vi "ReadMDF.vi"() -> (2 "Number of Waypoints Read":i32, 3 "MDF Array out":T2)   [LabVIEW 2010]
uses:
  4-High Neurons/MDFArray.ctl
  4-High Neurons/MissionDefinitionFile.ctl
panel:
  in  "MissionDefinition":T1={"Waypoint #"=2.0, "X (waypoint)"=0.0, "Y (waypoint)"=0.0, "Vel (desired)"=0.0, "Dwell Time"=0.0, "Behavior"=enum."OpenFieldTransit", "Expand1"=0.0, "Expand2"=0.0, "Expand3"=0.0}
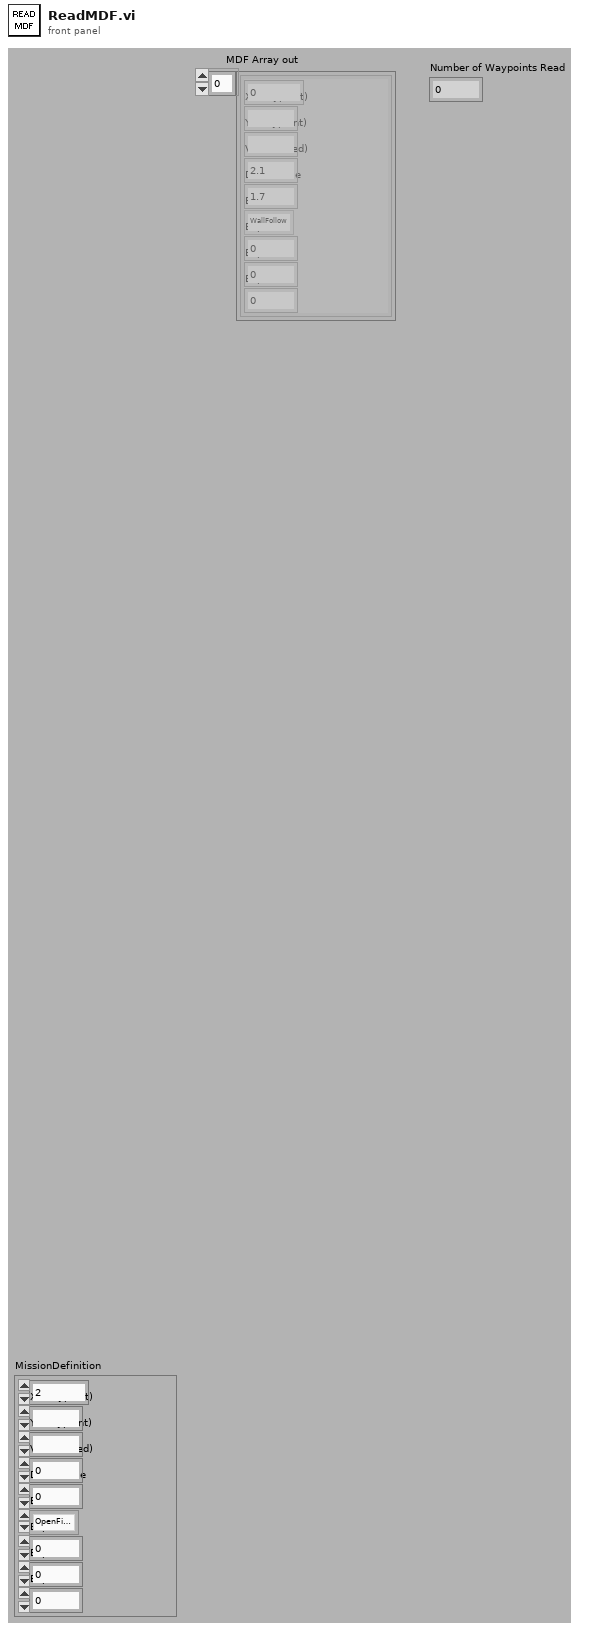
[diagram p1: front panel]
types:
  T1 = typedef "MissionDefinitionFile.ctl" = cluster{"Waypoint #":dbl, "X (waypoint)":ext, "Y (waypoint)":ext, "Vel (desired)":dbl, "Dwell Time":dbl, "Behavior":enum16{"OpenFieldTransit", "WallFollow", "LaneFollow", "ManualMode"}, "Expand1":dbl, "Expand2":dbl, "Expand3":dbl}
  T2 = typedef "MDFArray.ctl" = T1[]
  T3 = enum16{"open", "replace", "create", "open or create", "replace or create", "replace or create with confirmation"}
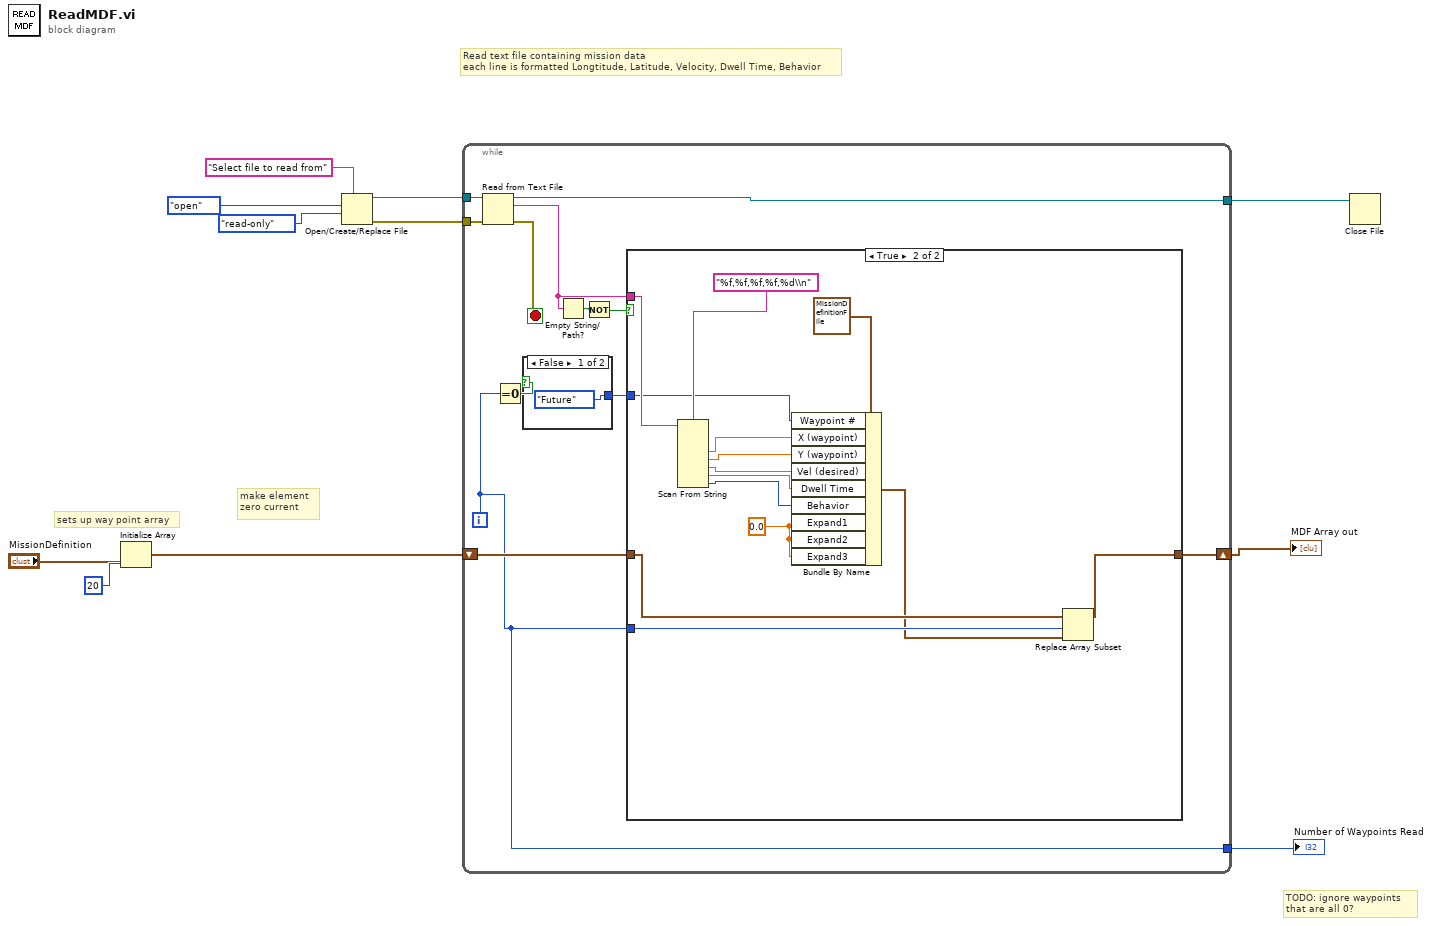
[diagram p0: block diagram]
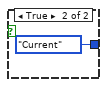
[diagram p2: hidden frame]
diagram:
  # "TODO: ignore waypoints \nthat are all 0?"
  # "Read text file containing mission data\neach line is formatted Longtitude, Latitude, Velocity, Dwell Time, Behavior"
  # "make element \nzero current"
  # "sets up way point array"
  n1 = Initialize Array ("Initialize WaypointArray")("MissionDefinition", 20 ("dimension size")) -> (w3:T1[])
  n2 = Open/Create/Replace File(prompt="Select file to read from", operation (0:open)=T3."open", access (0:read/write)=enum16{"read/write", "read-only", "write-only"}."read-only") -> (refnum out=w11:refnum<file>, error out=w6:errorcluster)  [unwired: 3 in, 1 out]
  n3 = while {
    tunnel: w11 -> [w23]
    tunnel: [w22] -> w10
    tunnel: w6 -> [w20]
    shift-right: [w16] -> w2
    shift-left: w3 -> [w15]
    tunnel: [w12] -> w1
    i -> [w12]
    stop <- w21 stop-if-true
    n4 = Read from Text File(file (use dialog)=w23, error in=w20) -> (refnum out=w22:refnum<file>, text=w17:string, error out=w21:errorcluster)  [unwired: 2 in, 1 out]
    n5 = Equal To 0?(x=w12) -> (x = 0?=w14:bool)
    n6 = case shown="False" w14 {
      tunnel: [enum16{"Past", "Current", "Future"}."Future" ("Status") enum16{"Past", "Current", "Future"}."Current" ("Status")] -> w13
      frame False {
      }
      frame True {
      }
    }
    n7 = Empty String/Path?(string/path=w17) -> (empty?=w19:bool)
    n8 = Not(x=w19) -> (.not. x?=w18:bool)
    n9 = case shown="True" w18 {
      tunnel: w17 -> [_ w39]
      tunnel: [w26 w30] -> w16
      tunnel: w15 -> [w26 w29]
      tunnel: w13 -> [_ w31]
      tunnel: w12 -> [_ w28]
      frame False {
      }
      frame True {
        w32 = 0.0 ("Expand1")
        n10 = Scan From String(format string="%f,%f,%f,%f,%d\\n", input string=w39) -> (output 1=w37:dbl, output 2=w36:dbl, output 3=w35:dbl, output 4=w34:dbl, output 5=w33:i32)  [unwired: 7 in, 3 out]
        n11 = Bundle By Name(cluster=T1 {"Waypoint #"=2.0, "X (waypoint)"=0.0, "Y (waypoint)"=0.0, "Vel (desired)"=0.0, "Dwell Time"=0.0, "Behavior"=enum."OpenFieldTransit", "Expand1"=0.0, "Expand2"=0.0, "Expand3"=0.0} ("MissionDefinitionFile"), "Waypoint #"=w31, "X (waypoint)"=w37, "Y (waypoint)"=w36, "Vel (desired)"=w35, "Dwell Time"=w34, "Behavior"=w33, "Expand1"=w32, "Expand2"=w32, "Expand3"=w32) -> (w27:T1)
        n12 = Replace Array Subset(array=w29, new element=w27, index=w28) -> (w30:T1[])
      }
    }
  }
  "MDF Array out" <- w2
  "Number of Waypoints Read" <- w1
  n13 = Close File(refnum=w10) -> ()  [unwired: 1 in, 2 out]
